vi "Collection.vi"(0 "Data":T2={"Message"="", "Freq."=0.0, "Collect Ref"=refnum, "Settings Ref"=refnum, "Data Display Ref"=refnum, "Exit Button Ref"=refnum, "Masking Ref"=refnum, "Calibrate Ref"=refnum, "Trial"=0, "Condition"="", "Subject"="", "Flow Feedback"=FALSE, "Audio Feedback"=FALSE, "All Data"=[], "Pressure/Flow"=[], "Audio"=[], "Flow Intercept"=0.0, " Flow Slope"=0.0, "Pressure Intercept"=0.0, "Pressure Slope"=0.0, "SGP Slope"=1.0, "SGP Intercept"=0.0, "Sex"=enum."Male", "Calibration Opened?"=FALSE, "Settings Opened?"=FALSE, "Test Type"=enum."Simulated", "Delay"=0, "Flow Array"=[], "Random Trials?"=FALSE, "Trials per condition"=0, "Condition/Trial Array"=[]}, 11 "Error In":errorcluster) -> (2 "Pulse 1":dbl, 6 "Save Data":dynamicdata(graph), 8 "Audio":dynamicdata(graph), 10 "Cancelled?":bool, 14 "Trial":i32, 15 "Error Out":errorcluster)   [LabVIEW 2020, in "CollectionSupport.lvlib"]
uses:
  CollectionSupport.lvlib
  Controls/UI Data.ctl
  Controls/Male_Female.ctl
  Controls/Test Type.ctl
  Controls/Collection States.ctl
  Controls/FirstCall.ctl
  <vilib>/Analysis/baseanly.llb/Mean (DBL).vi
  <vilib>/Analysis/NI_AALBase.lvlib
panel:
  in  "Time Target":dbl=6.0 format="%#_13g"
  out "Flow Chart":cluster{"Y":dbl[], "Y":dbl[]}[](graph)
  out "Condition":string
  out "Which Button?":T1(ring)
  out "Audio":dynamicdata(graph)
  out "SPL":dbl
  out "Airflow":dbl
  out "SPL Feedback Chart":dbl(graph)
  out "Pressure Chart":dynamicdata(graph)
  out "Flow Chart":dynamicdata(graph)
  out "Time Left":i32 caption="Elapsed Time (s)" format="%1.0f"
  # "Incomplete Interruption Testing"
  # "No Feedback Provided"
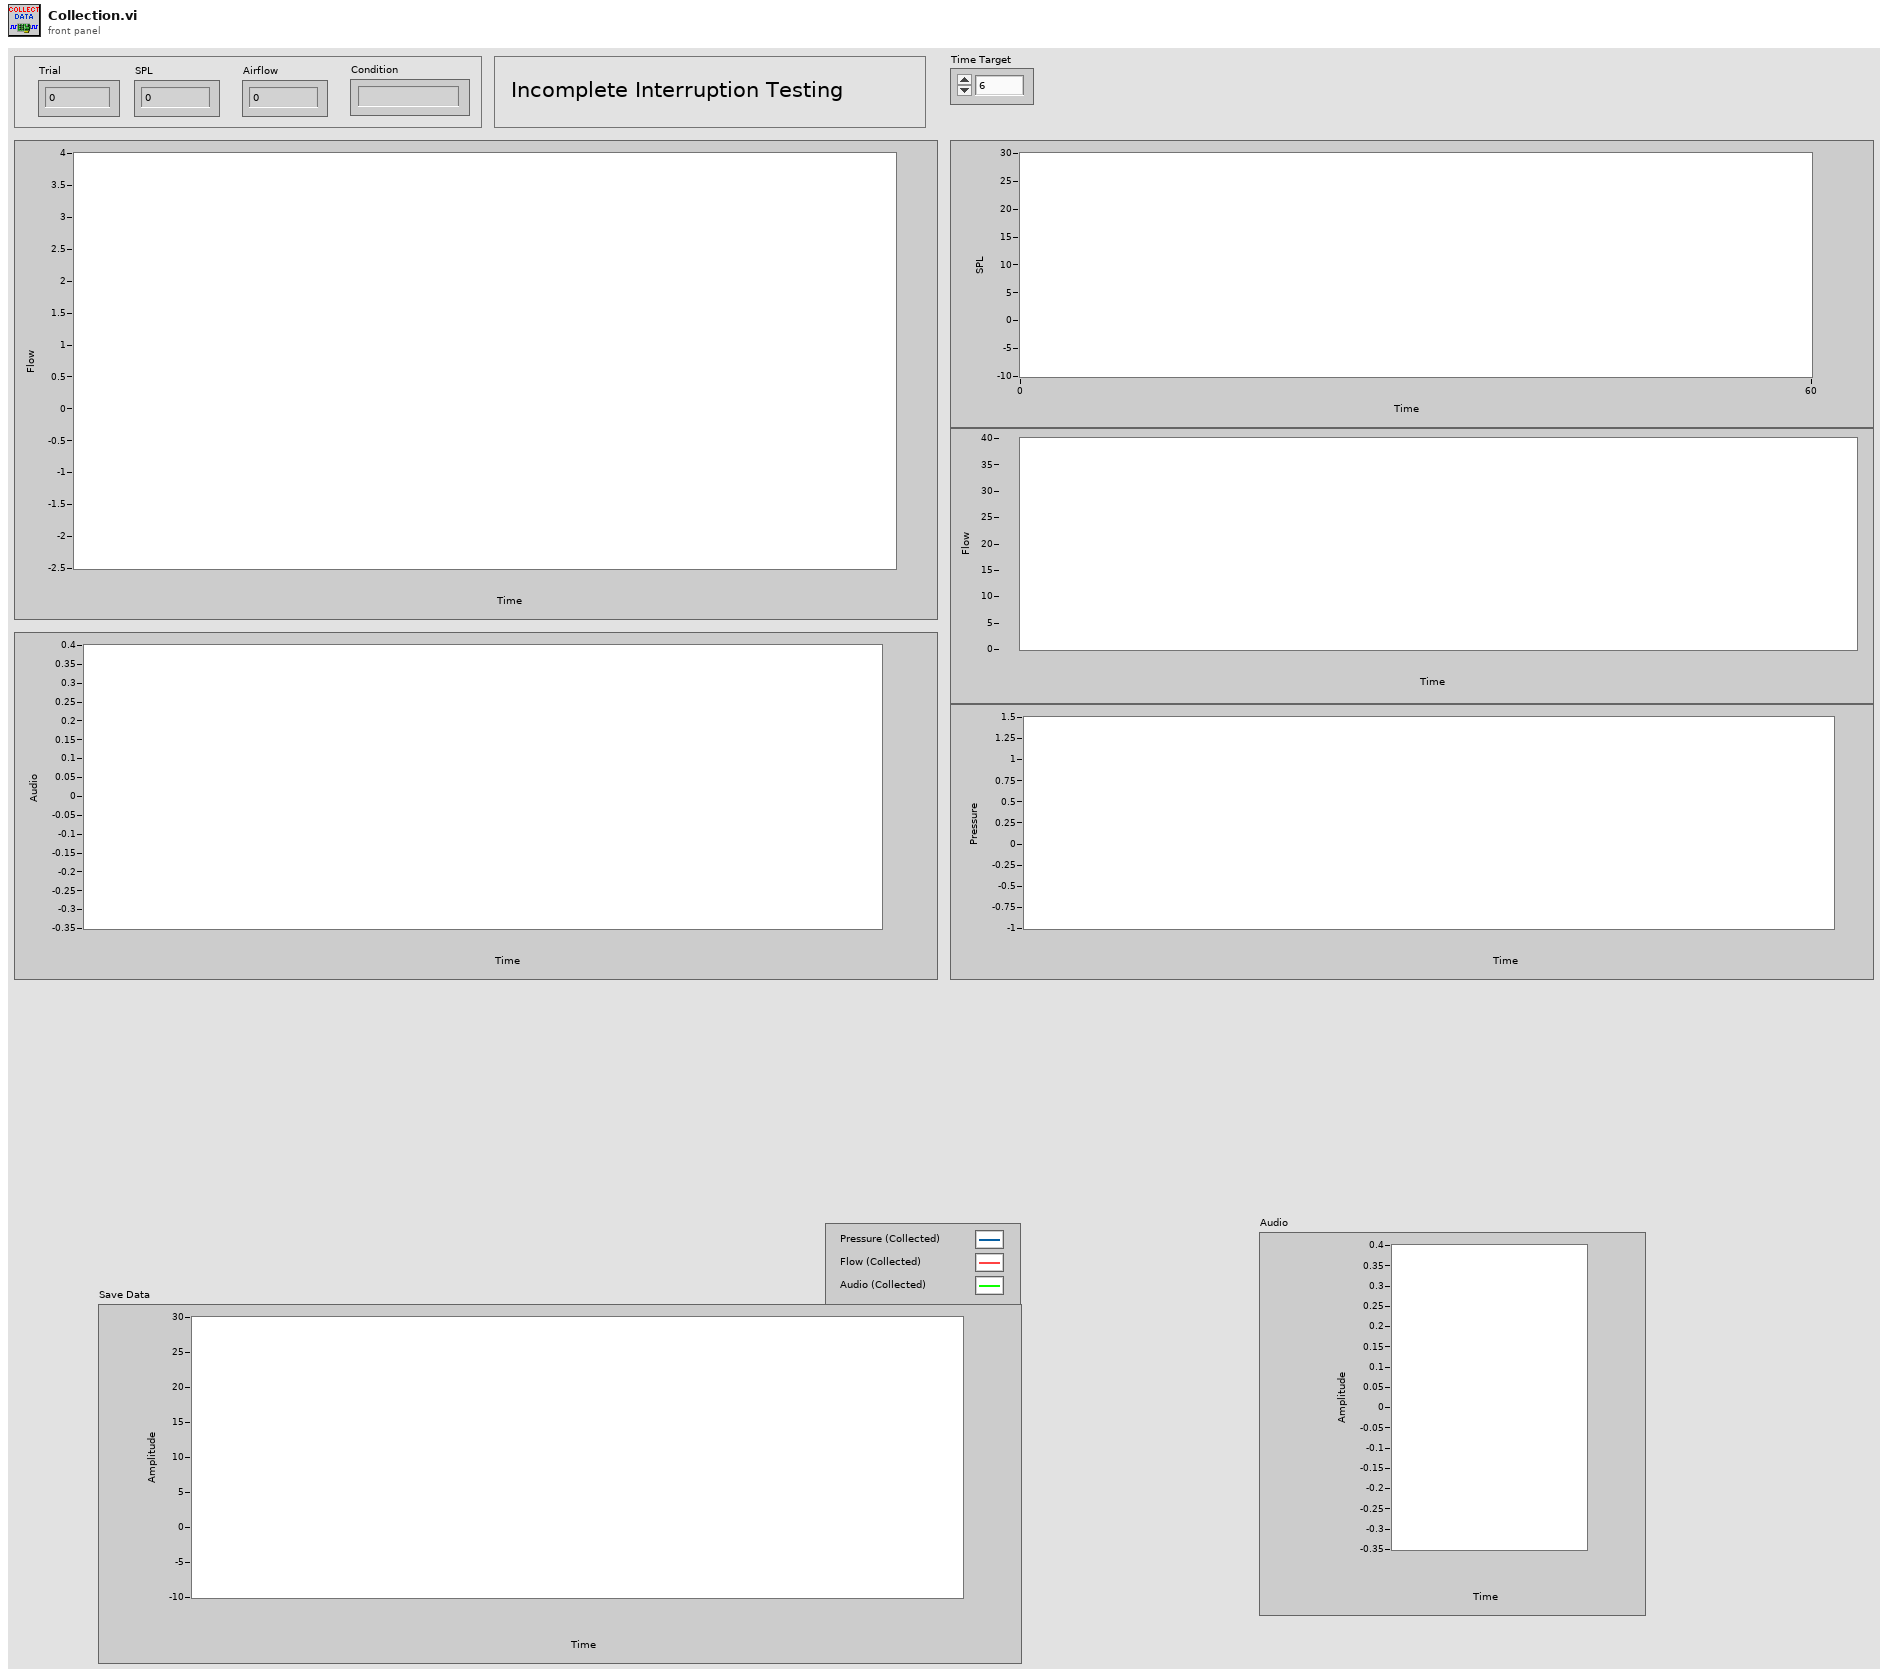
[diagram p1: front panel]
types:
  T1 = enum16{"Left Button", "Center Button", "Right Button", "Window Close"}
  T2 = typedef "CollectionSupport.lvlib/UI Data.ctl" = cluster{"Message":string, "Freq.":dbl, "Collect Ref":refnum<vi>, "Settings Ref":refnum<vi>, "Data Display Ref":refnum<vi>, "Exit Button Ref":refnum<vi>, "Masking Ref":refnum<vi>, "Calibrate Ref":refnum<vi>, "Trial":i32, "Condition":string, "Subject":string, "Flow Feedback":bool, "Audio Feedback":bool, "All Data":dynamicdata, "Pressure/Flow":dynamicdata, "Audio":dynamicdata, "Flow Intercept":dbl, " Flow Slope":dbl, "Pressure Intercept":dbl, "Pressure Slope":dbl, "SGP Slope":dbl, "SGP Intercept":dbl, "Sex":T3, "Calibration Opened?":bool, "Settings Opened?":bool, "Test Type":T4, "Delay":u32, "Flow Array":dbl[], "Random Trials?":bool, "Trials per condition":i32, "Condition/Trial Array":i32[]}
  T3 = typedef "CollectionSupport.lvlib/Male_Female.ctl" = enum16{"Female", "Male"}
  T4 = typedef "CollectionSupport.lvlib/Test Type.ctl" = enum32{"Simulated", "Human"}
  T5 = typedef "CollectionSupport.lvlib/Collection States.ctl" = enum16{"Start", "Run", "Check", "Exit"}
  T6 = typedef "CollectionSupport.lvlib/FirstCall.ctl" = enum16{"First", "After"}
  T7 = typedef "Sound Output Task ID.ctl" = u32
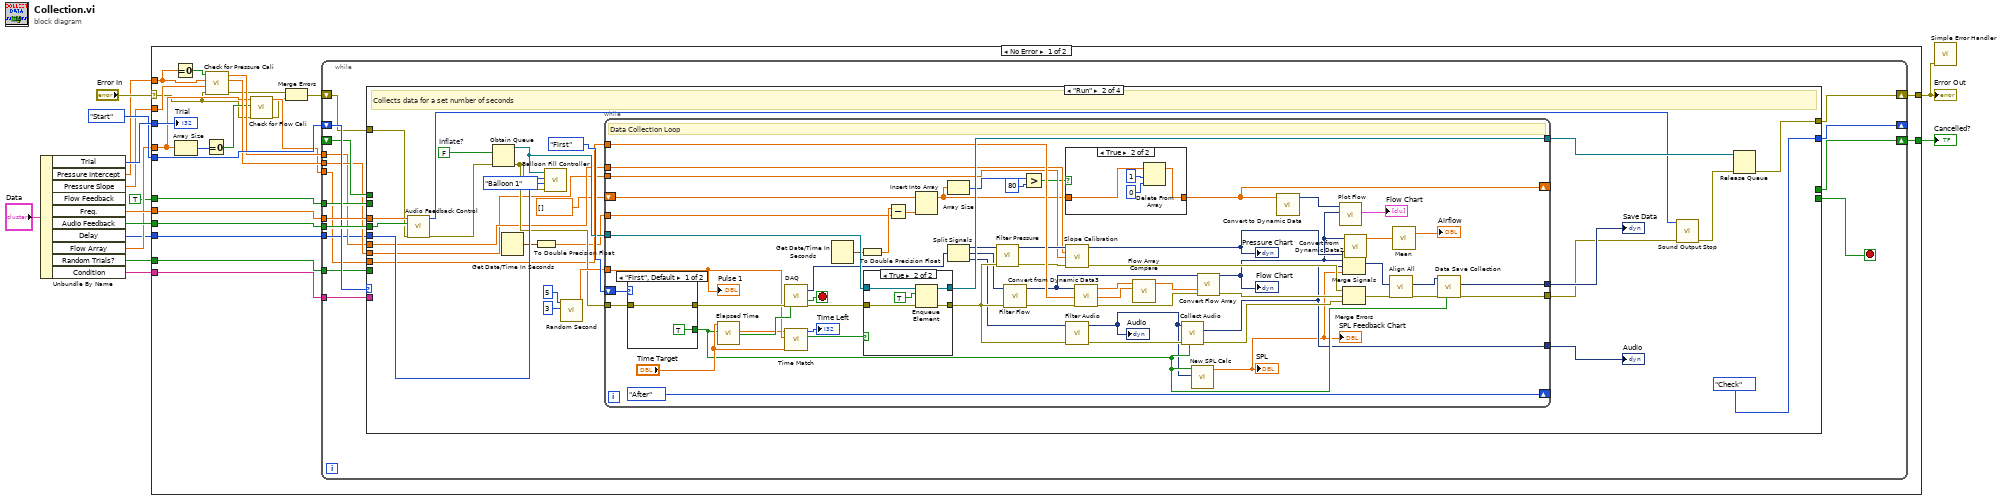
[diagram p0: block diagram]
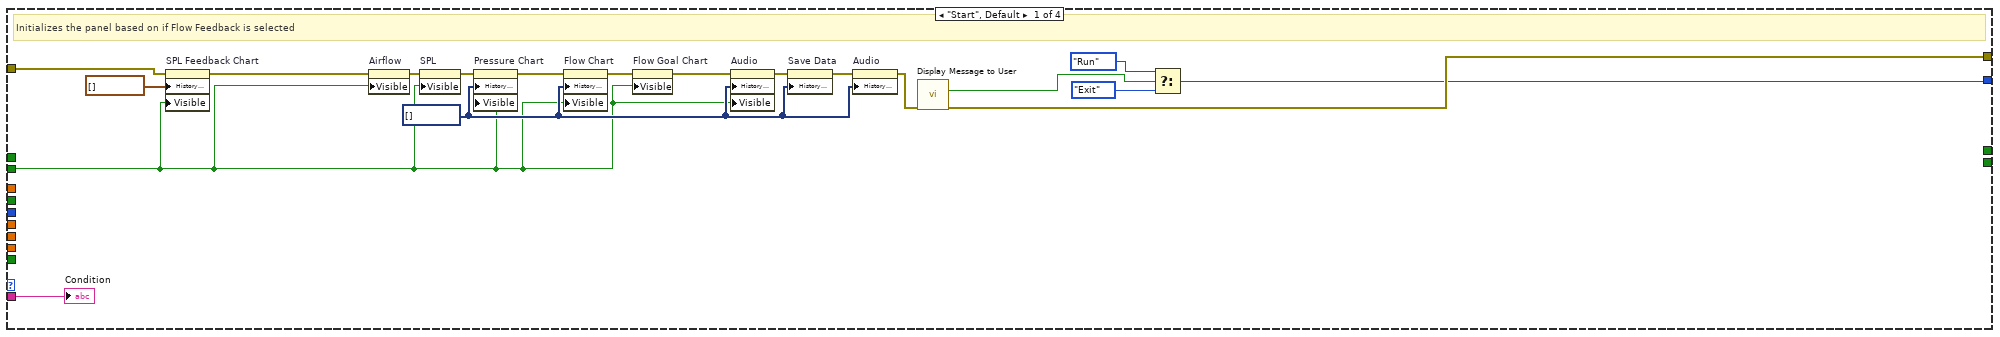
[diagram p2: hidden frame]
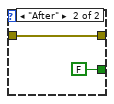
[diagram p5: hidden frame]
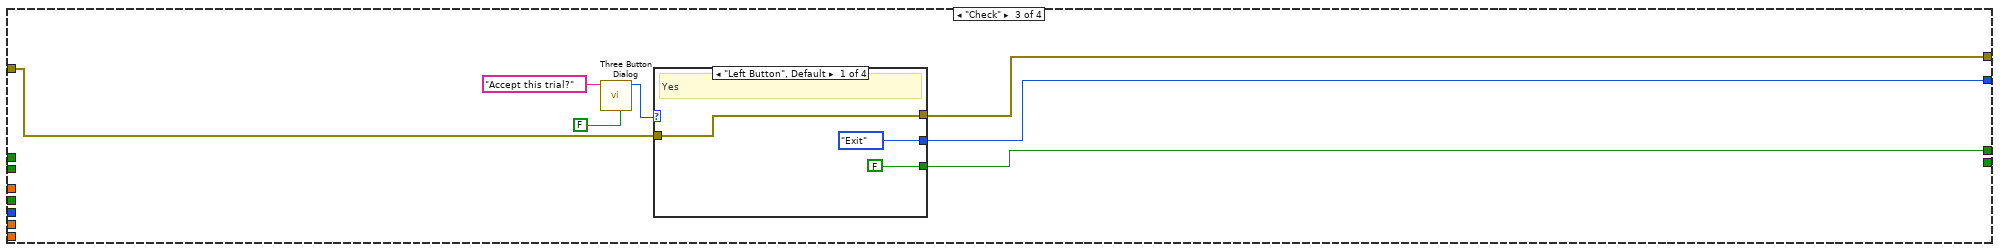
[diagram p6: hidden frame]
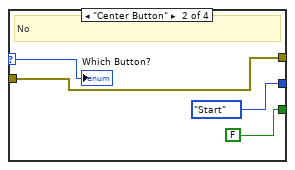
[diagram p7: hidden frame]
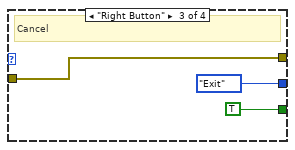
[diagram p8: hidden frame]
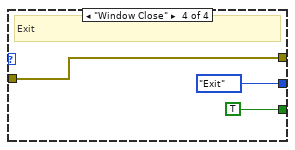
[diagram p9: hidden frame]
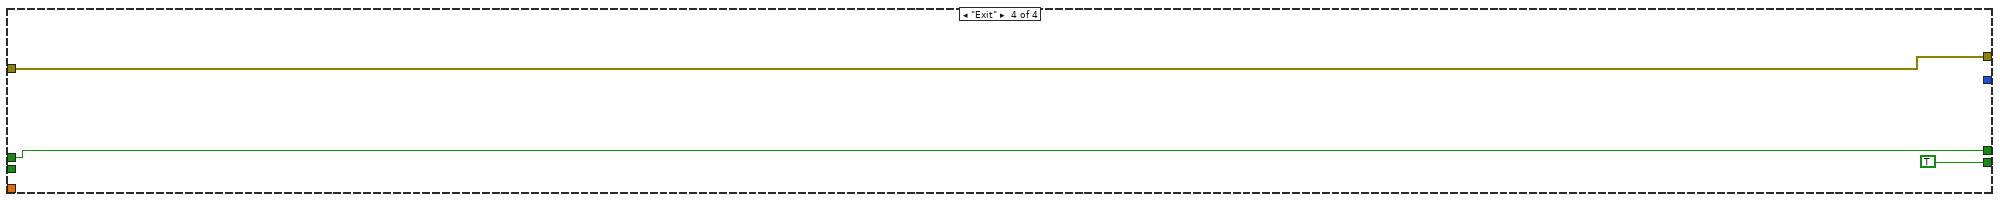
[diagram p10: hidden frame]
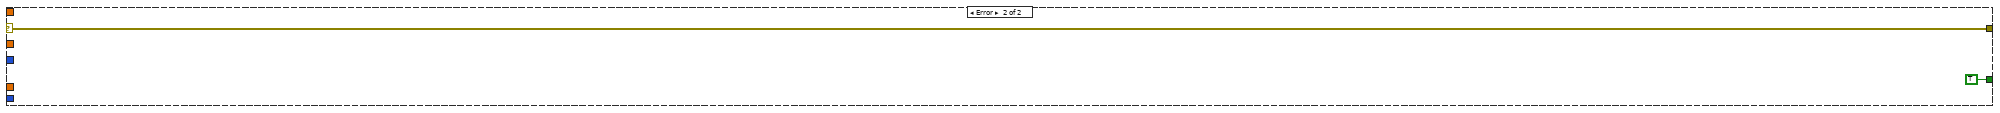
[diagram p11: hidden frame]
diagram:
  n1 = Unbundle By Name("Data") -> ("Trial"=w12:i32, "Pressure Intercept"=w10:dbl, "Pressure Slope"=w9:dbl, "Freq."=w8:dbl, "Audio Feedback"=w7:bool, "Delay"=w4:u32, "Flow Array"=w6:dbl[], "Random Trials?"=w3:bool, "Condition"=w2:string)  [unwired: 1 out]
  n2 = case shown="No Error" "Error In" {
    selector: "Error In" -> [w18 w199]
    tunnel: [w37 w199] -> w5
    tunnel: w8 -> [w38 _]
    tunnel: w12 -> [w36 _]
    tunnel: [w33 TRUE ("Allow user to close window? (TRUE)")] -> w14
    tunnel: w7 -> [w35 _]
    tunnel: Collection_States."Start" -> [w34 _]
    tunnel: TRUE -> [w32 _]
    tunnel: w10 -> [w29 _]
    tunnel: w9 -> [w27 _]
    tunnel: w4 -> [w31 _]
    tunnel: w6 -> [w21 _]
    tunnel: w3 -> [w17 _]
    tunnel: w2 -> [w16 _]
    frame No Error {
      n3 = Equal To 0?(x=w29) -> (x = 0?=w30:bool)
      n4 = Array Size(array=w21) -> (size(s)=w25:i32)
      n5 = Equal To 0?(x=w25) -> (x = 0?=w22:bool)
      n6 = call "Check for Pressure Cali.vi"("error in (no error)"=w18, "Pressure Slope in"=w27, "Pressure Intercept in"=w29, "Intercept and Slope available?"=w30) -> ("error out"=w23:errorcluster, "Pressure Intercept out"=w28:dbl, "Pressure Slope out"=w26:dbl)  [unwired: 5 in]
      n7 = call "Check for Flow Cali.vi"("error in (no error)"=w18, "Flow array available?"=w22, "Flow Array in"=w21) -> ("error out"=w19:errorcluster, "Flow Array out"=w20:dbl[])  [unwired: 7 in]
      n8 = Merge Errors(w23, w19) -> (w24:errorcluster)
      n9 = while {
        tunnel: w35 -> [w54]
        tunnel: w38 -> [w53]
        shift-right: [w49] -> _
        shift-left: w34 -> [w52]
        shift-right: [w51] -> w37
        shift-left: w24 -> [w50]
        tunnel: w32 -> [w46]
        shift-right: [w47] -> w33
        shift-left: _ -> [w45]
        tunnel: w28 -> [w44]
        tunnel: w26 -> [w43]
        tunnel: w31 -> [w42]
        tunnel: w20 -> [w41]
        tunnel: w17 -> [w40]
        tunnel: w16 -> [w39]
        stop <- w48 stop-if-true
        n10 = case shown="\"Run\"" w52 {
          tunnel: [w70 w89 w176 w196] -> w51
          tunnel: w54 -> [_ w100 _ _]
          tunnel: w53 -> [_ w99 _ _]
          tunnel: w50 -> [w61 w97 w177 w196]
          tunnel: [w67 Collection_States."Check" w178 _] -> w49
          tunnel: [_ _ _ TRUE] -> w48
          tunnel: [_ _ w175 w195] -> w47
          tunnel: w46 -> [w55 _ _ _]
          tunnel: w45 -> [_ _ _ w195]
          tunnel: w44 -> [_ w81 _ _]
          tunnel: w43 -> [_ w82 _ _]
          tunnel: w42 -> [_ w85 _ _]
          tunnel: w41 -> [_ w83 _ _]
          tunnel: w40 -> [_ _ _ _]
          tunnel: w39 -> [w60 _ _ _]
          frame "Start", Default {
            w57 = dynamicdata[] [] ("History Data")
            # "Initializes the panel based on if Flow Feedback is selected"
            n11 = property on="SPL Feedback Chart" class="WFChart (strict)"(error in=w61, "History Data"=waveform(dbl)[] [], "Visible"=w55) -> (error out=w65:errorcluster)  [unwired: 1 in, 1 out]
            n12 = property on="Airflow" class="DigNum (strict)"(error in=w65, "Visible"=w55) -> (error out=w73:errorcluster)  [unwired: 1 in, 1 out]
            n13 = property on="SPL" class="DigNum (strict)"(error in=w73, "Visible"=w55) -> (error out=w72:errorcluster)  [unwired: 1 in, 1 out]
            n14 = property on="Pressure Chart" class="WFChart (strict)"(error in=w72, "History Data"=w57, "Visible"=w55) -> (error out=w62:errorcluster)  [unwired: 1 in, 1 out]
            n15 = property on="Flow Chart" class="WFChart (strict)"(error in=w62, "History Data"=w57, "Visible"=w55) -> (error out=w58:errorcluster)  [unwired: 1 in, 1 out]
            n16 = property on="Flow Goal Chart" class="XYGraph (strict)"(error in=w58, "Visible"=w55) -> (error out=w56:errorcluster)  [unwired: 1 in, 1 out]
            n17 = property on="Audio" class="WFChart (strict)"(error in=w56, "History Data"=w57, "Visible"=w55) -> (error out=w63:errorcluster)  [unwired: 1 in, 1 out]
            n18 = property on="Save Data" class="WFChart (strict)"(error in=w63, "History Data"=w57) -> (error out=w66:errorcluster)  [unwired: 1 in, 1 out]
            n19 = property on="Audio" class="WFChart (strict)"(error in=w66, "History Data"=w57) -> (error out=w59:errorcluster)  [unwired: 1 in, 1 out]
            n20 = call "Display Message to User"("error in (no error)"=w59) -> ("error out"=w70:errorcluster, "Start"=w71:bool)  [unwired: 9 in]
            n21 = Select(t=Collection_States."Run", s=w71, f=Collection_States."Exit") -> (s? t:f=w67:T5)
            "Condition" <- w60
          }
          frame "Run" {
            w87 = FALSE  # Inflate?
            # "Collects data for a set number of seconds"
            n22 = call "Audio Feedback Control.vi"("error in (no error)"=w97, "Audio Feedback"=w100, "Freq."=w99) -> ("error out"=w90:errorcluster, "task ID out"=w78:T7)  [unwired: 7 in]
            n23 = Obtain Queue(element data type=w87, error in (no error)=w90) -> (queue out=w88:refnum<queue>, error out=w84:errorcluster)  [unwired: 3 in, 1 out]
            n24 = Get Date/Time In Seconds() -> (seconds since 1Jan1904=w77:timestamp)
            n25 = To Double Precision Float(number=w77) -> (double precision float=w76:dbl)
            n26 = call "Balloon Fill Controller.vi"("error in (no error)"=w84, "Balloon Select"=enum16{"Balloon 1", "Balloon 3", "Balloon 4"}."Balloon 1", "Delay"=w85, "Queue in"=w88) -> ()  [unwired: 8 in]
            n27 = call "Random Second.vi"("Min Second"=3, "Max Second"=5) -> ("Random Second"=w91:dbl)  [unwired: 9 in]
            n28 = while {
              tunnel: w84 -> [w154]
              tunnel: [w157] -> w96
              tunnel: [w115] -> w95
              shift-right: [FirstCall."After"] -> _
              shift-left: FirstCall."First" -> [w156]
              tunnel: w91 -> [w145]
              tunnel: w82 -> [w134]
              tunnel: w81 -> [w135]
              tunnel: w88 -> [w149]
              tunnel: [w147] -> w86
              tunnel: [w141] -> w80
              tunnel: w83 -> [w140]
              tunnel: w76 -> [w109]
              shift-right: [w102] -> _
              shift-left: dbl[] [] -> [w108]
              stop <- w151 stop-if-true
              # "Data Collection Loop"
              n29 = case shown="\"First\", Default" w156 {
                tunnel: [TRUE FALSE] -> w125
                tunnel: w154 -> [w171 w173]
                tunnel: [w171 w173] -> w153
                frame "First", Default {
                }
                frame "After" {
                }
              }
              n30 = call "Elapsed Time"("Time Target (s)"="Time Target", "Reset"=w125) -> ("Elapsed Time (s)"=w144:dbl, "Time has Elapsed"=w150:bool)  [unwired: 10 in, 6 out]
              n31 = call "DAQ"("error in"=w153, "stop (F)"=w150) -> ("data"=w130:dynamicdata, "stopped"=w151:bool, "error out"=w131:errorcluster)  [unwired: 14 in, 1 out]
              n32 = call "Time Match.vi"("Time Target"="Time Target", "Random Second"=w145, "Elapsed Time (s)"=w144) -> ("Matched?"=w148:bool, "Time Left"=→"Time Left":i32)  [unwired: 6 in, 1 out]
              n33 = Get Date/Time In Seconds() -> (seconds since 1Jan1904=w111:timestamp)
              n34 = To Double Precision Float(number=w111) -> (double precision float=w110:dbl)
              n35 = case shown="True" w148 {
                tunnel: w131 -> [w164 w170]
                tunnel: [w164 w167] -> w142
                tunnel: w149 -> [w165 w169]
                tunnel: [w165 w168] -> w147
                frame False {
                }
                frame True {
                  n36 = Enqueue Element(queue=w169, element=TRUE, error in (no error)=w170) -> (queue out=w168:refnum<queue>, error out=w167:errorcluster)  [unwired: 1 in, 1 out]
                }
              }
              n37 = Subtract(x=w110, y=w109) -> (x-y=w107:dbl)
              n38 = Insert Into Array(array=w108, new element=w107) -> (w103:dbl[])  [unwired: 1 in]
              n39 = Array Size(array=w103) -> (size(s)=w106:i32)
              n40 = Split Signals(w130) -> (w143:dynamicdata, w128:dynamicdata, w129:dynamicdata)  [unwired: 3 in]
              n41 = call "Filter Pressure"("error in (no error)"=w142, "Signal"=w143) -> ("error out"=w136:errorcluster, "Filtered Signal"=w137:dynamicdata)  [unwired: 8 in]
              n42 = call "Filter Flow"("error in (no error)"=w142, "Signal"=w128) -> ("error out"=w132:errorcluster, "Filtered Signal"=w127:dynamicdata)  [unwired: 8 in]
              n43 = Greater?(x=w106, y=80) -> (0:w104:bool)
              n44 = case shown="True" w104 {
                tunnel: w103 -> [w159 w163]
                tunnel: [w159 w162] -> w102
                frame False {
                }
                frame True {
                  n45 = Delete From Array(array=w163, length=1, index=0) -> (array with subset deleted=w162:dbl[])  [unwired: 1 out]
                }
              }
              n46 = call "Slope Calibration.vi"("Voltage"=w137, "Slope"=w134, "Intercept"=w135, "error in (no error)"=w136) -> ("Result"=w116:dynamicdata, "error out"=w120:errorcluster)  [unwired: 10 in]
              "Pressure Chart" <- w116
              n47 = call "Filter Audio"("error in (no error)"=w142, "Signal"=w129) -> ("error out"=w126:errorcluster, "Filtered Signal"=w117:dynamicdata)  [unwired: 8 in]
              "Audio" <- w117
              n48 = call "Convert from Dynamic Data3"("Dynamic Data Type"=w127) -> ("Array"=w139:dbl[])  [unwired: 3 in]
              n49 = call "Flow Array Compare.vi"("Flow Array in"=w140, "Array in"=w139) -> ("Array out"=w133:dbl[])  [unwired: 9 in]
              n50 = call "Collect Audio"("Reset"=w125, "error in (no error)"=w126, "Signals"=w117) -> ("error out"=w118:errorcluster, "Collected Signals"=w115:dynamicdata)  [unwired: 7 in]
              n51 = call "New SPL Calc.vi"("Filtered Signal"=w117, "Reset"=w125) -> ("SPL Out"=w114:dbl)  [unwired: 9 in]
              "SPL" <- w114
              "SPL Feedback Chart" <- w114
              n52 = call "Convert Flow Array.vi"("Voltage"=w127, "Array - Numeric"=w133, "error in (no error)"=w132) -> ("Result"=w112:dynamicdata, "error out"=w119:errorcluster)  [unwired: 11 in]
              "Flow Chart" <- w112
              n53 = call "Convert to Dynamic Data"("Array"=w102) -> ("Dynamic Data Type"=w101:dynamicdata)  [unwired: 3 in]
              n54 = call "Plot Flow"("Y Input"=w112, "X Input"=w101) -> ("XY Graph"=→"Flow Chart":cluster{"Y":dbl[], "Y":dbl[]}[])  [unwired: 8 in, 1 out]
              n55 = Merge Signals(w116, w112, w115, w114) -> (w124:dynamicdata)
              n56 = Merge Errors(w120, w119, w118) -> (w123:errorcluster)
              n57 = call "Convert from Dynamic Data2"("Dynamic Data Type"=w112) -> ("Array"=w158:dbl[])  [unwired: 3 in]
              n58 = call "Align All"("error in (no error)"=w123, "Signals"=w124) -> ("error out"=w122:errorcluster, "Resampled Signals"=w121:dynamicdata)  [unwired: 7 in, 1 out]
              n59 = call-poly <vilib>:"Mean.vi"("X"=w158) -> ("mean"=→"Airflow":dbl)  [unwired: 1 out]
              n60 = call "Data Save Collection"("Reset"=w125, "error in (no error)"=w122, "Signals"=w121) -> ("error out"=w141:errorcluster, "Collected Signals"=w157:dynamicdata)  [unwired: 7 in]
              "Pulse 1" <- w145
            }
            "Save Data" <- w96
            "Audio" <- w95
            n61 = call <vilib>:"Sound Output Stop.vi"("error in (no error)"=w80, "task ID"=w78) -> ("error out"=w79:errorcluster)  [unwired: 8 in, 1 out]
            n62 = Release Queue(queue=w86, error in (no error)=w79) -> (error out=w89:errorcluster)  [unwired: 1 in, 2 out]
          }
          frame "Check" {
            n63 = call <vilib>:"Three Button Dialog.vi"("Allow user to close window? (TRUE)"=FALSE, "message"="Accept this trial?") -> ("Which Button?"=w180:T1)  [unwired: 9 in]
            n64 = case shown="\"Left Button\", Default" w180 {
              selector: w180 -> [_ w185 _ _]
              tunnel: [FALSE ("Allow user to close window? (TRUE)") FALSE ("Allow user to close window? (TRUE)") TRUE TRUE ("Allow user to close window? (TRUE)")] -> w175
              tunnel: [Collection_States."Exit" Collection_States."Start" Collection_States."Exit" Collection_States."Exit"] -> w178
              tunnel: w177 -> [w183 w187 w190 w192]
              tunnel: [w183 w187 w190 w192] -> w176
              frame "Left Button", Default {
                # "Yes"
              }
              frame "Center Button" {
                # "No"
                "Which Button?" <- w185
              }
              frame "Right Button" {
                # "Cancel"
              }
              frame "Window Close" {
                # "Exit"
              }
            }
          }
          frame "Exit" {
          }
        }
      }
      "Trial" <- w36
    }
    frame Error {
    }
  }
  "Error Out" <- w5
  "Cancelled?" <- w14
  n65 = call <vilib>:"Simple Error Handler.vi"("error in (no error)"=w5) -> ()  [unwired: 4 in, 5 out]
